vi "Get Header Strings.vi"(11 "CSV Settings":T1) -> (3 "Header Values":string[](array[string]))   [LabVIEW 2022 SP3, in "CSV Export.lvlib" / "CSV Export.lvclass"]
uses:
  CSV Export.lvclass
  Controls/CSV Export Settings.ctl
  CSV Export.lvclass/CSV Export.ctl
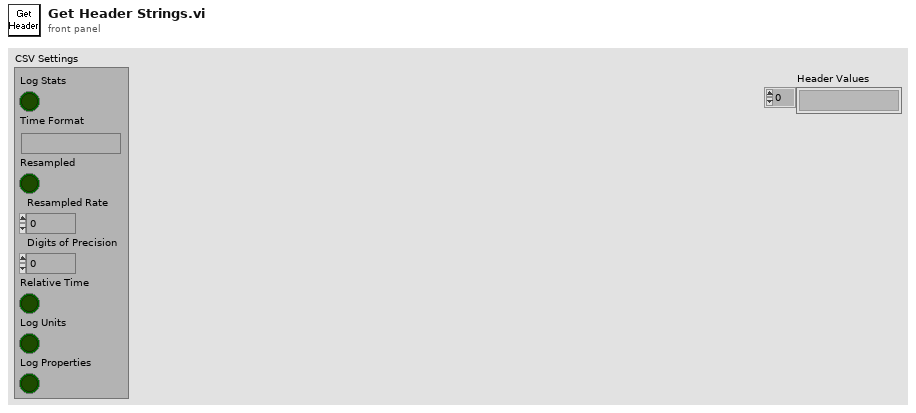
[diagram p1: front panel]
types:
  T1 = typedef "CSV Export.lvlib/CSV Export.lvclass/CSV Export Settings.ctl" = cluster{"Log Stats":bool, "Time Format":string, "Resampled":bool, "Resampled Rate":dbl, "Digits of Precision":u32, "Relative Time":bool, "Log Units":bool, "Log Properties":bool}
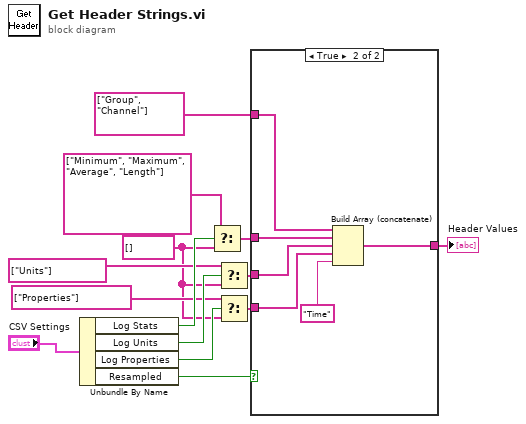
[diagram p0: block diagram]
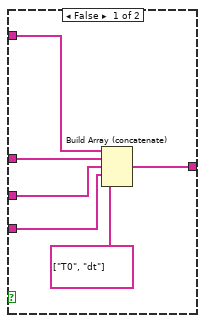
[diagram p2: hidden frame]
diagram:
  w2 = string[] []
  n1 = Unbundle By Name("CSV Settings") -> ("Log Stats"=w10:bool, "Log Units"=w9:bool, "Log Properties"=w4:bool, "Resampled"=w5:bool)
  n2 = Select(t=string[] ["Minimum", "Maximum", "Average", "Length"], s=w10, f=w2) -> (s? t:f=w12:string[])
  n3 = Select(t=string[] ["Units"], s=w9, f=w2) -> (s? t:f=w8:string[])
  n4 = Select(t=string[] ["Properties"], s=w4, f=w2) -> (s? t:f=w1:string[])
  n5 = case shown="True" w5 {
    tunnel: string[] ["Group", "Channel"] -> [w20 w26]
    tunnel: w12 -> [w19 w25]
    tunnel: [w18 w24] -> w11
    tunnel: w8 -> [w17 w23]
    tunnel: w1 -> [w16 w22]
    frame False {
      n6 = Build Array (concatenate)(w20, w19, w17, w16, string[] ["T0", "dt"]) -> (w18:string[])
    }
    frame True {
      n7 = Build Array (concatenate)(w26, w25, w23, w22, "Time") -> (w24:string[])
    }
  }
  "Header Values" <- w11
